vi "JSON Parse Array.vi"(8 "error in (no error)":errorcluster, 10 "JSON Array Value":string="[{\"Numeric\":121,\"Boolean\":false,\"Enum\":\"first\",\"Path\":\"C:\\test\",\"String\":\"examplestring\"},{\"Numeric\":121,\"Boolean\":true,\"Enum\":\"second\",\"Path\":\"D:\\stest\",\"String\":\"asdfasd\"}]", 11 "Type":variant=variant(cluster{"Numeric":dbl, "Boolean":bool, "Enum":enum16{"first", "second"}, "Path":path, "String":string}[] [{"Numeric"=121.0, "Boolean"=FALSE, "Enum"=enum."first", "Path"=path "C:/test", "String"="examplestring"}, {"Numeric"=121.0, "Boolean"=TRUE, "Enum"=enum."second", "Path"=path "D:/stest", "String"="asdfasd"}])) -> (0 "error out":errorcluster, 1 "JSON type":T2, 3 "variant":variant, 5 "Type Enum":T1)   [LabVIEW 2013, in "LV JSON.lvlib"]
doc: "Separate array elements and output in string representation. Also output the JSON type for validation."
uses:
  LV JSON.lvlib
  controls/JSON type.ctl
  <vilib>/Utility/VariantDataType/Type.ctl
  JSON Type.vi
  <vilib>/Utility/error.llb/Trim Whitespace.vi
  <vilib>/Utility/VariantDataType/VariantType.lvlib
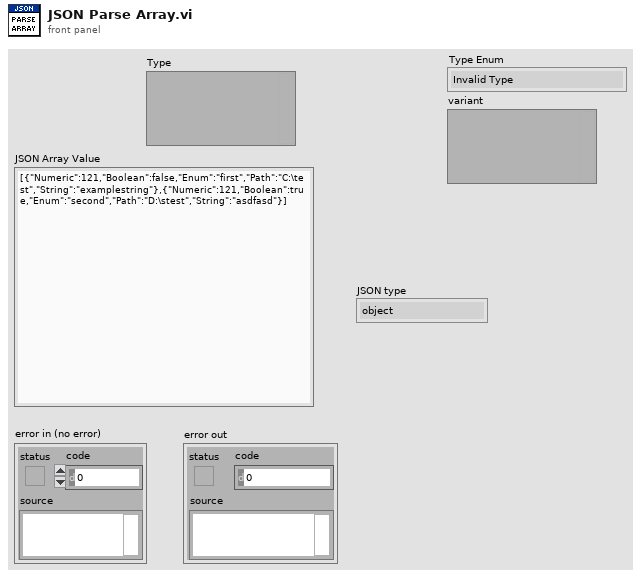
[diagram p1: front panel]
types:
  T1 = typedef "VariantType.lvlib/Type.ctl" = enum8{"Invalid Type", "Void", "I8", "I16", "I32", "I64", "U8", "U16", "U32", "U64", "Single Float", "Double Float", "Extended Float", "Single Complex", "Double Complex", "Extended Complex", "Enum U8", "Enum U16", "Enum U32", "Enum U64", "Single Float With Unit", "Double Float With Unit", "Extended Float With Unit", "Single Complex with Unit", "Double Complex with Unit", "Extended Complex with Unit", "Boolean", "String", "Path", "Picture", "Tag", "Array", "Cluster", "Variant", "LV Variant", "Waveform", "Timestamp", "Digital Waveform", "Digital Data", "ExpressData", "Refnum", "External Data", "VI", "Poly VI", "LabVIEW Class Instance", "Fixed Point"}
  T2 = typedef "LV JSON.lvlib/JSON type.ctl" = enum16{"object", "array", "number", "string", "boolean", "null"}
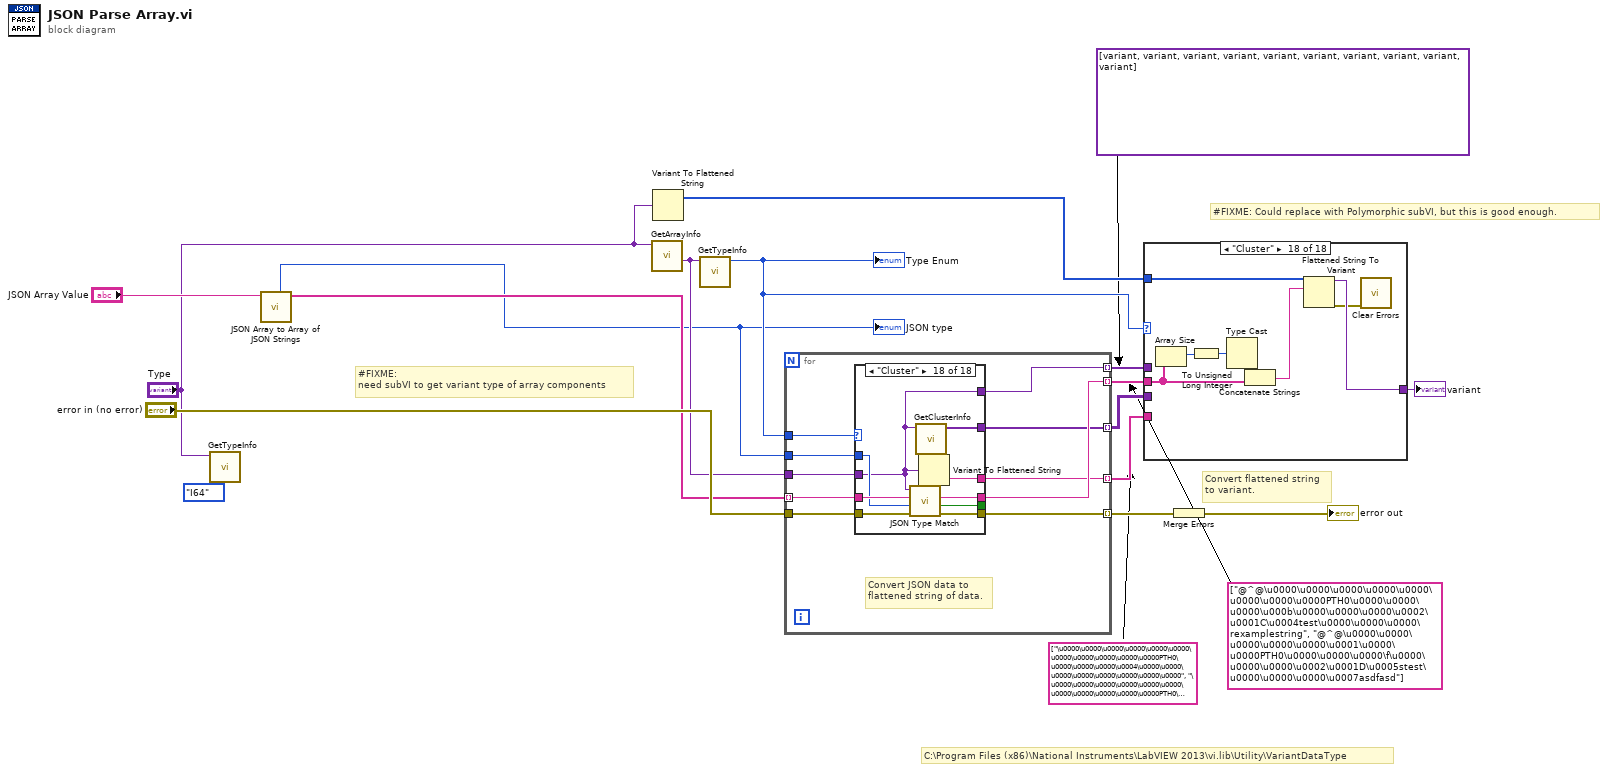
[diagram p0: block diagram]
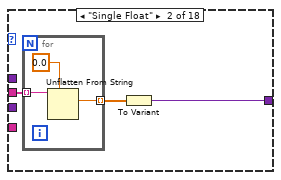
[diagram p3: hidden frame]
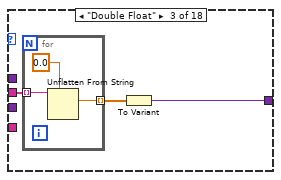
[diagram p4: hidden frame]
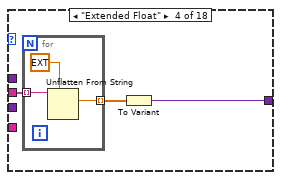
[diagram p5: hidden frame]
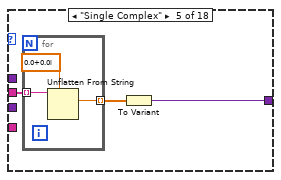
[diagram p6: hidden frame]
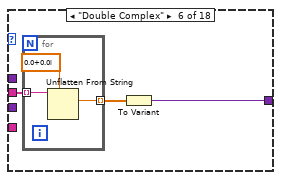
[diagram p7: hidden frame]
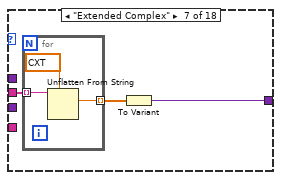
[diagram p8: hidden frame]
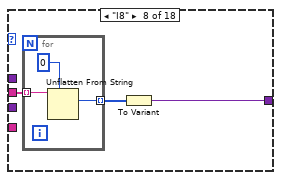
[diagram p9: hidden frame]
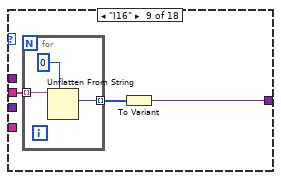
[diagram p10: hidden frame]
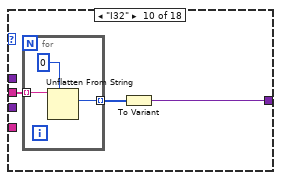
[diagram p11: hidden frame]
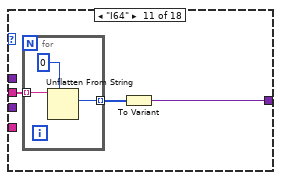
[diagram p12: hidden frame]
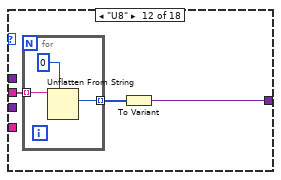
[diagram p13: hidden frame]
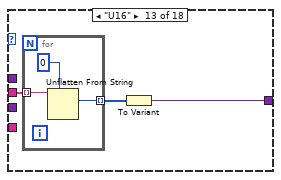
[diagram p14: hidden frame]
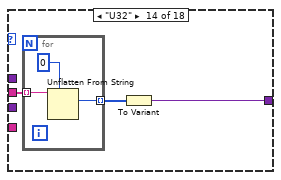
[diagram p15: hidden frame]
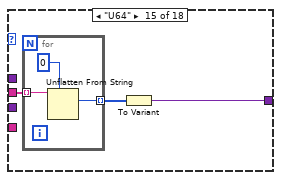
[diagram p16: hidden frame]
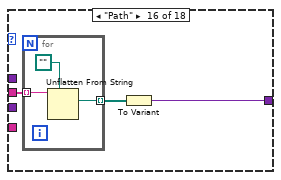
[diagram p17: hidden frame]
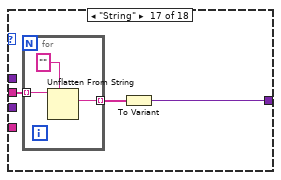
[diagram p18: hidden frame]
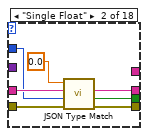
[diagram p20: hidden frame]
diagram:
  (unwired) string[] ["\u0000\u0000\u0000\u0000\u0000\u0000\u0000\u0000\u0000\u0000\u0000PTH0\u0000\u0000\u0000\u0004\u0000\u0000\u0000\u0000\u0000\u0000\u0000\u0000", "\u0000\u0000\u0000\u0000\u0000\u0000\u0000\u0000\u0000\u0000\u0000PTH0\u0000\u0000\u0000\u0004\u0000\u0000\u0000\u0000\u0000\u0000\u0000\u0000"]
  (unwired) string[] ["@^@\u0000\u0000\u0000\u0000\u0000\u0000\u0000\u0000PTH0\u0000\u0000\u0000\u000b\u0000\u0000\u0000\u0002\u0001C\u0004test\u0000\u0000\u0000\rexamplestring", "@^@\u0000\u0000\u0000\u0000\u0000\u0001\u0000\u0000PTH0\u0000\u0000\u0000\f\u0000\u0000\u0000\u0002\u0001D\u0005stest\u0000\u0000\u0000\u0007asdfasd"]
  (unwired) variant[][] [[variant(dbl 0.0), variant(bool FALSE), variant(enum16{"first", "second"} enum."first"), variant(path path ""), variant(string "")], [variant(dbl 0.0), variant(bool FALSE), variant(enum16{"first", "second"} enum."first"), variant(path path ""), variant(string "")]] ("Cluster Elements")
  (unwired) Type."I64" ("Type Enum")
  # "Convert flattened string\nto variant."
  # "#FIXME: Could replace with Polymorphic subVI, but this is good enough."
  # "C:\\Program Files (x86)\\National Instruments\\LabVIEW 2013\\vi.lib\\Utility\\VariantDataType"
  # "#FIXME:\nneed subVI to get variant type of array components"
  n1 = call <vilib>:"GetTypeInfo.vi"("Variant"="Type") -> ()  [unwired: 6 in, 5 out]
  n2 = call "JSON Array to Array of JSON Strings.vi"("JSON Array Value"="JSON Array Value") -> ("Array of JSON Values"=w4:string[], "JSON Value Type"=w3:T2)  [unwired: 9 in]
  "JSON type" <- w3
  n3 = call <vilib>:"GetArrayInfo.vi"("Variant"="Type") -> ("ArrayElement"=w14:variant)  [unwired: 7 in, 3 out]
  n4 = Variant To Flattened String(Variant="Type") -> (1:w1:i16[])  [unwired: 1 out]
  n5 = call <vilib>:"GetTypeInfo.vi"("Variant"=w14) -> ("Type Enum"=w11:T1)  [unwired: 6 in, 4 out]
  "Type Enum" <- w11
  n6 = for {
    tunnel: w4 -> [w24] mode=indexing
    tunnel: w3 -> [w22]
    tunnel: "error in (no error)" -> [w23]
    tunnel: w14 -> [w19]
    tunnel: w11 -> [w25]
    tunnel: [w21] -> w13 mode=indexing
    tunnel: [w20] -> w6 mode=indexing
    tunnel: [w18] -> w9 mode=indexing
    tunnel: [w17] -> w8 mode=indexing
    tunnel: [w16] -> w7 mode=indexing
    # "Convert JSON data to\nflattened string of data."
    n7 = case shown="\"Cluster\"" w25 {
      tunnel: w24 -> [_ w32 w39 w46 w53 w60 w67 w74 w81 w88 w95 w102 w109 w116 w123 w130 w137 w146]
      tunnel: w23 -> [_ w31 w38 w45 w52 w59 w66 w73 w80 w87 w94 w101 w108 w115 w122 w129 w136 w145]
      tunnel: w22 -> [_ w30 w37 w44 w51 w58 w65 w72 w79 w86 w93 w100 w107 w114 w121 w128 w135 w144]
      tunnel: [_ w28 w35 w42 w49 w56 w63 w70 w77 w84 w91 w98 w105 w112 w119 w126 w133 w143] -> w20
      tunnel: [_ w27 w34 w41 w48 w55 w62 w69 w76 w83 w90 w97 w104 w111 w118 w125 w132 w142] -> _
      tunnel: [_ w26 w33 w40 w47 w54 w61 w68 w75 w82 w89 w96 w103 w110 w117 w124 w131 w141] -> w21
      tunnel: w19 -> [_ _ _ _ _ _ _ _ _ _ _ _ _ _ _ _ _ w138]
      tunnel: [_ _ _ _ _ _ _ _ _ _ _ _ _ _ _ _ _ w140] -> w17
      tunnel: [_ _ _ _ _ _ _ _ _ _ _ _ _ _ _ _ _ w139] -> w18
      tunnel: [_ _ _ _ _ _ _ _ _ _ _ _ _ _ _ _ _ w138] -> w16
      frame "Invalid Type", Default {
      }
      frame "Single Float" {
        n8 = call "JSON Type Match.vi"("error in (no error)"=w31, "JSON Type"=w30, "JSON Value"=w32, "Type"=sgl 0.0) -> ("error out"=w26:errorcluster, "Types Match"=w27:bool, "Variant Data String"=w28:string)  [unwired: 5 in]
      }
      frame "Double Float" {
        n9 = call "JSON Type Match.vi"("error in (no error)"=w38, "JSON Type"=w37, "JSON Value"=w39, "Type"=0.0) -> ("error out"=w33:errorcluster, "Types Match"=w34:bool, "Variant Data String"=w35:string)  [unwired: 5 in]
      }
      frame "Extended Float" {
        n10 = call "JSON Type Match.vi"("error in (no error)"=w45, "JSON Type"=w44, "JSON Value"=w46, "Type"=ext 0.0) -> ("error out"=w40:errorcluster, "Types Match"=w41:bool, "Variant Data String"=w42:string)  [unwired: 5 in]
      }
      frame "I8" {
        n11 = call "JSON Type Match.vi"("error in (no error)"=w52, "JSON Type"=w51, "JSON Value"=w53, "Type"=i8 0) -> ("error out"=w47:errorcluster, "Types Match"=w48:bool, "Variant Data String"=w49:string)  [unwired: 5 in]
      }
      frame "I16" {
        n12 = call "JSON Type Match.vi"("error in (no error)"=w59, "JSON Type"=w58, "JSON Value"=w60, "Type"=i16 0) -> ("error out"=w54:errorcluster, "Types Match"=w55:bool, "Variant Data String"=w56:string)  [unwired: 5 in]
      }
      frame "I32" {
        n13 = call "JSON Type Match.vi"("error in (no error)"=w66, "JSON Type"=w65, "JSON Value"=w67, "Type"=0) -> ("error out"=w61:errorcluster, "Types Match"=w62:bool, "Variant Data String"=w63:string)  [unwired: 5 in]
      }
      frame "I64" {
        n14 = call "JSON Type Match.vi"("error in (no error)"=w73, "JSON Type"=w72, "JSON Value"=w74, "Type"=i64 0) -> ("error out"=w68:errorcluster, "Types Match"=w69:bool, "Variant Data String"=w70:string)  [unwired: 5 in]
      }
      frame "U8" {
        n15 = call "JSON Type Match.vi"("error in (no error)"=w80, "JSON Type"=w79, "JSON Value"=w81, "Type"=u8 0) -> ("error out"=w75:errorcluster, "Types Match"=w76:bool, "Variant Data String"=w77:string)  [unwired: 5 in]
      }
      frame "U16" {
        n16 = call "JSON Type Match.vi"("error in (no error)"=w87, "JSON Type"=w86, "JSON Value"=w88, "Type"=u16 0) -> ("error out"=w82:errorcluster, "Types Match"=w83:bool, "Variant Data String"=w84:string)  [unwired: 5 in]
      }
      frame "U32" {
        n17 = call "JSON Type Match.vi"("error in (no error)"=w94, "JSON Type"=w93, "JSON Value"=w95, "Type"=u32 0) -> ("error out"=w89:errorcluster, "Types Match"=w90:bool, "Variant Data String"=w91:string)  [unwired: 5 in]
      }
      frame "U64" {
        n18 = call "JSON Type Match.vi"("error in (no error)"=w101, "JSON Type"=w100, "JSON Value"=w102, "Type"=u64 0) -> ("error out"=w96:errorcluster, "Types Match"=w97:bool, "Variant Data String"=w98:string)  [unwired: 5 in]
      }
      frame "Single Complex" {
        n19 = call "JSON Type Match.vi"("error in (no error)"=w108, "JSON Type"=w107, "JSON Value"=w109, "Type"=csg 0.0+0.0i) -> ("error out"=w103:errorcluster, "Types Match"=w104:bool, "Variant Data String"=w105:string)  [unwired: 5 in]
      }
      frame "Double Complex" {
        n20 = call "JSON Type Match.vi"("error in (no error)"=w115, "JSON Type"=w114, "JSON Value"=w116, "Type"=cdb 0.0+0.0i) -> ("error out"=w110:errorcluster, "Types Match"=w111:bool, "Variant Data String"=w112:string)  [unwired: 5 in]
      }
      frame "Extended Complex" {
        n21 = call "JSON Type Match.vi"("error in (no error)"=w122, "JSON Type"=w121, "JSON Value"=w123, "Type"=cxt 0.0+0.0i) -> ("error out"=w117:errorcluster, "Types Match"=w118:bool, "Variant Data String"=w119:string)  [unwired: 5 in]
      }
      frame "Path" {
        n22 = call "JSON Type Match.vi"("error in (no error)"=w129, "JSON Type"=w128, "JSON Value"=w130, "Type"=path "") -> ("error out"=w124:errorcluster, "Types Match"=w125:bool, "Variant Data String"=w126:string)  [unwired: 5 in]
      }
      frame "String" {
        n23 = call "JSON Type Match.vi"("error in (no error)"=w136, "JSON Type"=w135, "JSON Value"=w137, "Type"="") -> ("error out"=w131:errorcluster, "Types Match"=w132:bool, "Variant Data String"=w133:string)  [unwired: 5 in]
      }
      frame "Cluster" {
        n24 = call "JSON Type Match.vi"("error in (no error)"=w145, "JSON Type"=w144, "JSON Value"=w146, "Type"=w138) -> ("error out"=w141:errorcluster, "Types Match"=w142:bool, "Variant Data String"=w143:string)  [unwired: 5 in]
        n25 = call <vilib>:"GetClusterInfo.vi"("Variant"=w138) -> ("Cluster Elements"=w140:variant[])  [unwired: 9 in, 1 out]
        n26 = Variant To Flattened String(Variant=w138) -> (data string=w139:string)  [unwired: 1 out]
      }
    }
  }
  n27 = case shown="\"Cluster\"" w11 {
    tunnel: w6 -> [_ w149 w155 w161 w167 w173 w179 w185 w191 w197 w203 w209 w215 w221 w227 w233 w239 w248]
    tunnel: [_ w147 w153 w159 w165 w171 w177 w183 w189 w195 w201 w207 w213 w219 w225 w231 w237 w244] -> w10
    tunnel: w9 -> [_ _ _ _ _ _ _ _ _ _ _ _ _ _ _ _ _ _]
    tunnel: w8 -> [_ _ _ _ _ _ _ _ _ _ _ _ _ _ _ _ _ _]
    tunnel: w7 -> [_ _ _ _ _ _ _ _ _ _ _ _ _ _ _ _ _ _]
    tunnel: w1 -> [_ _ _ _ _ _ _ _ _ _ _ _ _ _ _ _ _ w246]
    frame "Invalid Type", Default {
    }
    frame "Single Float" {
      n28 = for {
        tunnel: w149 -> [w151] mode=indexing
        tunnel: [w150] -> w148 mode=indexing
        n29 = Unflatten From String(type=sgl 0.0, binary string=w151) -> (value=w150:sgl)  [unwired: 3 in, 2 out]
      }
      n30 = To Variant(anything=w148) -> (Variant=w147:variant)
    }
    frame "Double Float" {
      n31 = for {
        tunnel: w155 -> [w157] mode=indexing
        tunnel: [w156] -> w154 mode=indexing
        n32 = Unflatten From String(type=0.0, binary string=w157) -> (value=w156:dbl)  [unwired: 3 in, 2 out]
      }
      n33 = To Variant(anything=w154) -> (Variant=w153:variant)
    }
    frame "Extended Float" {
      n34 = for {
        tunnel: w161 -> [w163] mode=indexing
        tunnel: [w162] -> w160 mode=indexing
        n35 = Unflatten From String(type=ext 0.0, binary string=w163) -> (value=w162:ext)  [unwired: 3 in, 2 out]
      }
      n36 = To Variant(anything=w160) -> (Variant=w159:variant)
    }
    frame "Single Complex" {
      n37 = for {
        tunnel: w167 -> [w169] mode=indexing
        tunnel: [w168] -> w166 mode=indexing
        n38 = Unflatten From String(type=csg 0.0+0.0i, binary string=w169) -> (value=w168:csg)  [unwired: 3 in, 2 out]
      }
      n39 = To Variant(anything=w166) -> (Variant=w165:variant)
    }
    frame "Double Complex" {
      n40 = for {
        tunnel: w173 -> [w175] mode=indexing
        tunnel: [w174] -> w172 mode=indexing
        n41 = Unflatten From String(type=cdb 0.0+0.0i, binary string=w175) -> (value=w174:cdb)  [unwired: 3 in, 2 out]
      }
      n42 = To Variant(anything=w172) -> (Variant=w171:variant)
    }
    frame "Extended Complex" {
      n43 = for {
        tunnel: w179 -> [w181] mode=indexing
        tunnel: [w180] -> w178 mode=indexing
        n44 = Unflatten From String(type=cxt 0.0+0.0i, binary string=w181) -> (value=w180:cxt)  [unwired: 3 in, 2 out]
      }
      n45 = To Variant(anything=w178) -> (Variant=w177:variant)
    }
    frame "I8" {
      n46 = for {
        tunnel: w185 -> [w187] mode=indexing
        tunnel: [w186] -> w184 mode=indexing
        n47 = Unflatten From String(type=i8 0, binary string=w187) -> (value=w186:i8)  [unwired: 3 in, 2 out]
      }
      n48 = To Variant(anything=w184) -> (Variant=w183:variant)
    }
    frame "I16" {
      n49 = for {
        tunnel: w191 -> [w193] mode=indexing
        tunnel: [w192] -> w190 mode=indexing
        n50 = Unflatten From String(type=i16 0, binary string=w193) -> (value=w192:i16)  [unwired: 3 in, 2 out]
      }
      n51 = To Variant(anything=w190) -> (Variant=w189:variant)
    }
    frame "I32" {
      n52 = for {
        tunnel: w197 -> [w199] mode=indexing
        tunnel: [w198] -> w196 mode=indexing
        n53 = Unflatten From String(type=0, binary string=w199) -> (value=w198:i32)  [unwired: 3 in, 2 out]
      }
      n54 = To Variant(anything=w196) -> (Variant=w195:variant)
    }
    frame "I64" {
      n55 = for {
        tunnel: w203 -> [w205] mode=indexing
        tunnel: [w204] -> w202 mode=indexing
        n56 = Unflatten From String(type=i64 0, binary string=w205) -> (value=w204:i64)  [unwired: 3 in, 2 out]
      }
      n57 = To Variant(anything=w202) -> (Variant=w201:variant)
    }
    frame "U8" {
      n58 = for {
        tunnel: w209 -> [w211] mode=indexing
        tunnel: [w210] -> w208 mode=indexing
        n59 = Unflatten From String(type=u8 0, binary string=w211) -> (value=w210:u8)  [unwired: 3 in, 2 out]
      }
      n60 = To Variant(anything=w208) -> (Variant=w207:variant)
    }
    frame "U16" {
      n61 = for {
        tunnel: w215 -> [w217] mode=indexing
        tunnel: [w216] -> w214 mode=indexing
        n62 = Unflatten From String(type=u16 0, binary string=w217) -> (value=w216:u16)  [unwired: 3 in, 2 out]
      }
      n63 = To Variant(anything=w214) -> (Variant=w213:variant)
    }
    frame "U32" {
      n64 = for {
        tunnel: w221 -> [w223] mode=indexing
        tunnel: [w222] -> w220 mode=indexing
        n65 = Unflatten From String(type=u32 0, binary string=w223) -> (value=w222:u32)  [unwired: 3 in, 2 out]
      }
      n66 = To Variant(anything=w220) -> (Variant=w219:variant)
    }
    frame "U64" {
      n67 = for {
        tunnel: w227 -> [w229] mode=indexing
        tunnel: [w228] -> w226 mode=indexing
        n68 = Unflatten From String(type=u64 0, binary string=w229) -> (value=w228:u64)  [unwired: 3 in, 2 out]
      }
      n69 = To Variant(anything=w226) -> (Variant=w225:variant)
    }
    frame "Path" {
      n70 = for {
        tunnel: w233 -> [w235] mode=indexing
        tunnel: [w234] -> w232 mode=indexing
        n71 = Unflatten From String(type=path "", binary string=w235) -> (value=w234:path)  [unwired: 3 in, 2 out]
      }
      n72 = To Variant(anything=w232) -> (Variant=w231:variant)
    }
    frame "String" {
      n73 = for {
        tunnel: w239 -> [w241] mode=indexing
        tunnel: [w240] -> w238 mode=indexing
        n74 = Unflatten From String(type="", binary string=w241) -> (value=w240:string)  [unwired: 3 in, 2 out]
      }
      n75 = To Variant(anything=w238) -> (Variant=w237:variant)
    }
    frame "Cluster" {
      n76 = Array Size(array=w248) -> (size(s)=w249:i32)
      n77 = To Unsigned Long Integer(number=w249) -> (unsigned 32bit integer=w250:u32)
      n78 = Type Cast(x=w250) -> (*(type *) &x=w247:string)  [unwired: 1 in]
      n79 = Concatenate Strings(w247, w248) -> (w245:string)
      n80 = Flattened String To Variant(6:w245, 7:w246) -> (0:w243:errorcluster, 3:w244:variant)  [unwired: 1 in]
      n81 = call <vilib>:"Clear Errors.vi"("error in (no error)"=w243) -> ()  [unwired: 6 in, 1 out]
    }
  }
  "variant" <- w10
  n82 = Merge Errors(w13) -> (→"error out":errorcluster)
